vi "CR-字符串检测衬丝.vi"(8 "error in (no error)":errorcluster caption="错误输入（无错误）", 11 "名称或相对路径":string="Template Program") -> (0 "error in (no error) 2":errorcluster caption="错误输入（无错误）")   [LabVIEW 2017]
uses:
  Picture/SaveButtom.ctl
  <vilib>/vision/Measure.llb/Edge Options.ctl
  <vilib>/vision/Measure.llb/Edge Polarity.ctl
  <vilib>/userdefined/High Color/IMAQdx.ctl
  Global System.vi
  <vilib>/Utility/xml.llb/Write to XML File(string).vi
panel:
  in  "Line3 保护套基准ROI":bool
  in  "ROI获取 2":bool
  in  "line2 ROI获取":bool
  in  "line1 ROI获取":bool
  in  "相机选择":T1="cam4" caption="Session Out CCD3"
  in  "获取图像":bool
  in  "ROI获取":bool
  in  "保存图像":bool
  out "添加的路径":path
  in  "刷新":bool
  in  "测试按钮":bool
  in  "保存按钮":bool
  in  "Main":enum32{"主参数", "模板匹配参数 ", "ROI参数", "测试效果"}(tab)
  in  "衬丝检测基础参数":T2={"IsNorImage"=TRUE, "Exposure Values"=100289, "ImagePath"=path "C:/Users/hedongpo/Desktop/514-hdp/Alignment Assemble System/Test Picture/B/3.bmp"} caption="参数界面" {"Exposure Values" scale=0.0..200000.0}
  in  "CR- 衬丝检测参数":T6={"Settings (Clamp (Rake) 1)"={"Contrast"=65, "Filter width"=3, "Steepness"=6, "Subsampling Ratio"=9, "Show Search Area"=TRUE, "Show Search Lines"=FALSE, "Show Edges Found"=FALSE, "Show Result"=TRUE}, "Options (Find Straight Edge 1)"={"Search Direction"=0, "Edge Options"={"Edge Polarity"=1, "Kernel Size"=13, "Width"=1, "Minimum Edge Strength"=25.0, "Interpolation Type"=enum."Bilinear Fixed", "Data Processing Method"=enum."Average"}, "Show Search Area"=FALSE, "Show Search Lines"=FALSE, "Show Edges Found"=FALSE, "Show Result"=FALSE, "Search Area Color"=65280, "Search Lines Color"=255, "Edge Locations Color"=16776960, "Result Color"=16711680, "Overlay Group Name"=""}, "相对距离设定"={"上限"=925.0, "下限"=3.0}, "保护套角度"={"上限"=0.0, "下限"=0.0}, "保护套直径设定"={"上限"=0.0, "下限"=0.0}, "Edge Options (Edge Detector 1)"={"Edge Polarity"=0, "Kernel Size"=3, "Width"=3, "Minimum Edge Strength"=10.0, "Interpolation Type"=enum."Bilinear Fixed", "Data Processing Method"=enum."Average"}, "保护套标准位置"={"Start X"=0, "Start Y"=0, "End X"=0, "End Y"=0}} {"保护套标准位置"."Start X" scale=0.0..1024.0; "保护套标准位置"."End X" scale=0.0..1024.0; "Edge Options (Edge Detector 1)"."Edge Polarity" items=["All Edges", "Rising Edges", "Falling Edges"]; "Options (Find Straight Edge 1)"."Search Direction" items=["Left to Right", "Right to Left", "Top to Bottom", "Bottom to Top"]; "Options (Find Straight Edge 1)"."Edge Options"."Edge Polarity" items=["All Edges", "Rising Edges", "Falling Edges"]; "Options (Find Straight Edge 1)"."Edge Options"."Minimum Edge Strength" format="%.2f"; "Options (Find Straight Edge 1)"."Edge Options"."Width" step=2; "Options (Find Straight Edge 1)"."Edge Options"."Kernel Size" step=2}
  in  "CR- 衬丝检测ROI参数":T8 {"Line 2"."Start X" scale=0.0..1024.0; "Line 2"."End X" scale=0.0..1024.0; "clamp Rectangle"."Rotation" min=-90.0 max=90.0 step=1.0 format="%.2f"; "clamp Rectangle"."Left" scale=0.0..1024.0; "clamp Rectangle"."Right" scale=0.0..1024.0; "Line 1"."Start X" scale=0.0..1024.0; "Line 1"."End X" scale=0.0..1024.0; "find straight edge Rectangle"."Rotation" min=-90.0 max=90.0 step=1.0 format="%.2f"; "find straight edge Rectangle"."Left" scale=0.0..1024.0; "find straight edge Rectangle"."Right" scale=0.0..1024.0}
  out "保护套距离":bool
  out "原始图像":T9(plugin-control)
  out "Distance":sgl format="%.2f"
  out "衬丝有无":bool
  out "保护套与基准位置差异":sgl
  out "保护套直径":sgl
  out "路径输出":path
  in  "Vision Paramter Save Buttom":T10
  out "system time":string
  in  "取消按钮":bool
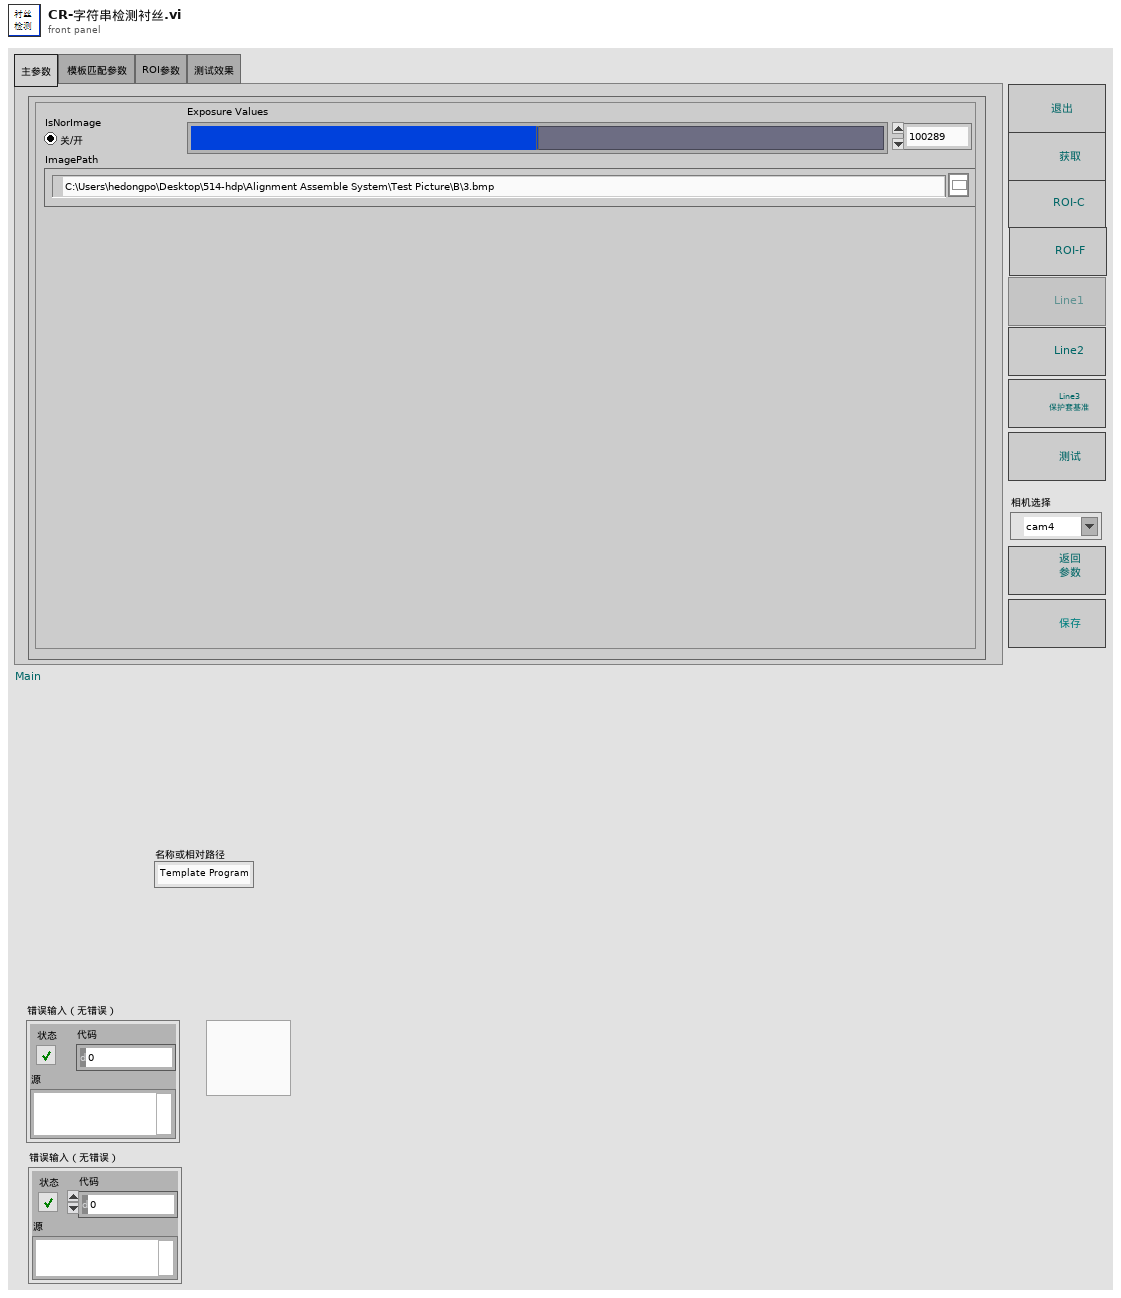
[diagram p1: front panel]
types:
  T1 = typedef "IMAQdx.ctl" = refnum<k21>
  T2 = cluster{"IsNorImage":bool, "Exposure Values":u32, "ImagePath":path}
  T3 = typedef "Edge Options.ctl" = cluster{"Edge Polarity":T4, "Kernel Size":u32, "Width":u32, "Minimum Edge Strength":sgl, "Interpolation Type":enum32{"Zero Order", "Bilinear", "Quadratic", "Cubic", "Bilinear Fixed"}, "Data Processing Method":enum32{"Average", "Median"}}
  T4 = typedef "Edge Polarity.ctl" = u32
  T5 = typedef "IMAQ Line" = cluster{"Start X":i32, "Start Y":i32, "End X":i32, "End Y":i32}
  T6 = cluster{"Settings (Clamp (Rake) 1)":cluster{"Contrast":i32, "Filter width":i32, "Steepness":i32, "Subsampling Ratio":u32, "Show Search Area":bool, "Show Search Lines":bool, "Show Edges Found":bool, "Show Result":bool}, "Options (Find Straight Edge 1)":cluster{"Search Direction":u32, "Edge Options":T3, "Show Search Area":bool, "Show Search Lines":bool, "Show Edges Found":bool, "Show Result":bool, "Search Area Color":u32, "Search Lines Color":u32, "Edge Locations Color":u32, "Result Color":u32, "Overlay Group Name":string}, "相对距离设定":cluster{"上限":dbl, "下限":dbl}, "保护套角度":cluster{"上限":dbl, "下限":dbl}, "保护套直径设定":cluster{"上限":dbl, "下限":dbl}, "Edge Options (Edge Detector 1)":cluster{"Edge Polarity":u32, "Kernel Size":u32, "Width":u32, "Minimum Edge Strength":sgl, "Interpolation Type":enum32{"Zero Order", "Bilinear", "Quadratic", "Cubic", "Bilinear Fixed"}, "Data Processing Method":enum32{"Average", "Median"}}, "保护套标准位置":T5}
  T7 = typedef "IMAQ Rectangle" = cluster{"Left":i32, "Top":i32, "Right":i32, "Bottom":i32, "Rotation":dbl}
  T8 = cluster{"find straight edge Rectangle":T7, "Line 1":T5, "clamp Rectangle ":T7, "Line 2":T5}
  T9 = typedef "IMAQ Image.ctl" = refnum<image>
  T10 = typedef "SaveButtom.ctl" = bool
  T11 = cluster{"index":i32, "this vi":refnum<vi>, "error out":errorcluster}
  T12 = cluster{"master data":string, "priority":u16, "secondary data":string[]}
  T13 = cluster{"case name":string[], "queue array":refnum<queue>[]}
  T14 = cluster{"Settings (Clamp (Rake) 1)":cluster{"Contrast":i32, "Filter width":i32, "Steepness":i32, "Subsampling Ratio":u32, "Show Search Area":bool, "Show Search Lines":bool, "Show Edges Found":bool, "Show Result":bool}, "Options (Find Straight Edge 1)":cluster{"Search Direction":u32, "Edge Options":T3, "Show Search Area":bool, "Show Search Lines":bool, "Show Edges Found":bool, "Show Result":bool, "Search Area Color":u32, "Search Lines Color":u32, "Edge Locations Color":u32, "Result Color":u32, "Overlay Group Name":string}, "相对距离设定":cluster{"上限":dbl, "下限":dbl}, "衬丝直径设定":cluster{"上限":dbl, "下限":dbl}, "保护套直径设定":cluster{"上限":dbl, "下限":dbl}, "Edge Options (Edge Detector 1)":cluster{"Edge Polarity":u32, "Kernel Size":u32, "Width":u32, "Minimum Edge Strength":sgl, "Interpolation Type":enum32{"Zero Order", "Bilinear", "Quadratic", "Cubic", "Bilinear Fixed"}, "Data Processing Method":enum32{"Average", "Median"}}, "保护套标准位置":T5}
  T15 = cluster{"Global Rectangle":i32[], "Contours":cluster{"Contour Type":u32, "ROI Type":u32, "Points":i32[]}[]}
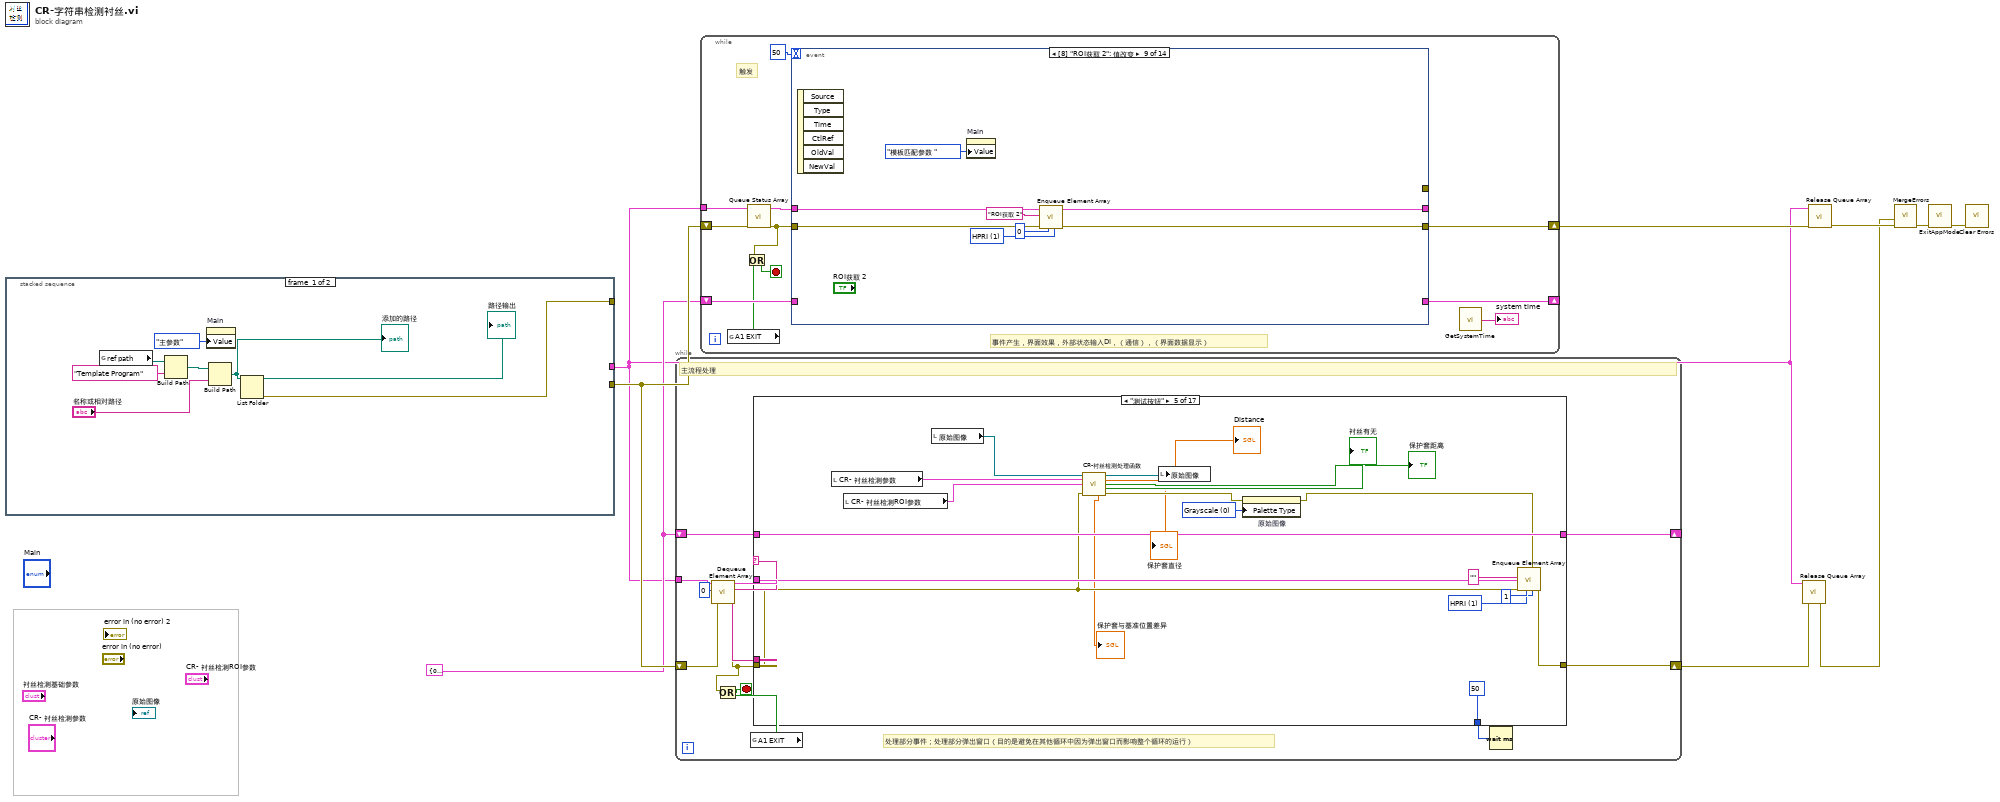
[diagram p0: block diagram]
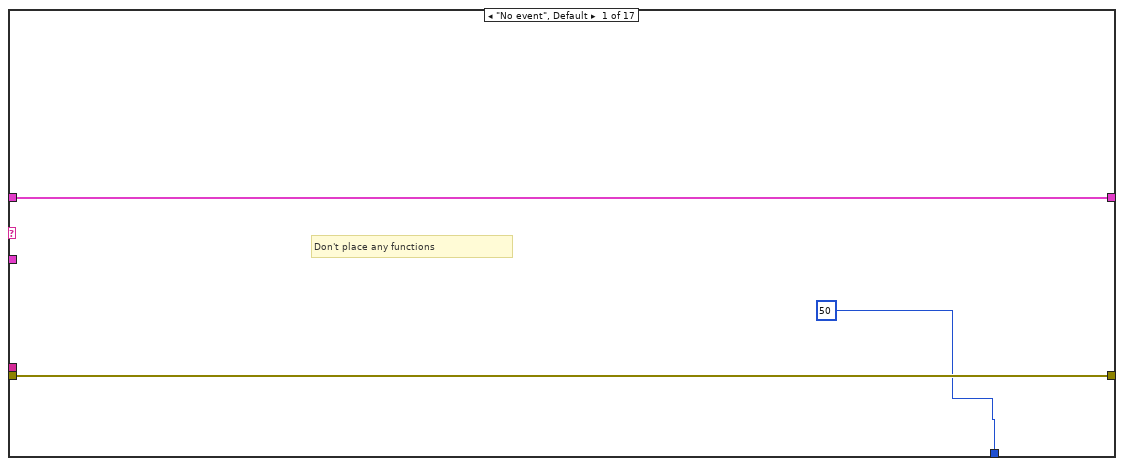
[diagram p2: hidden frame]
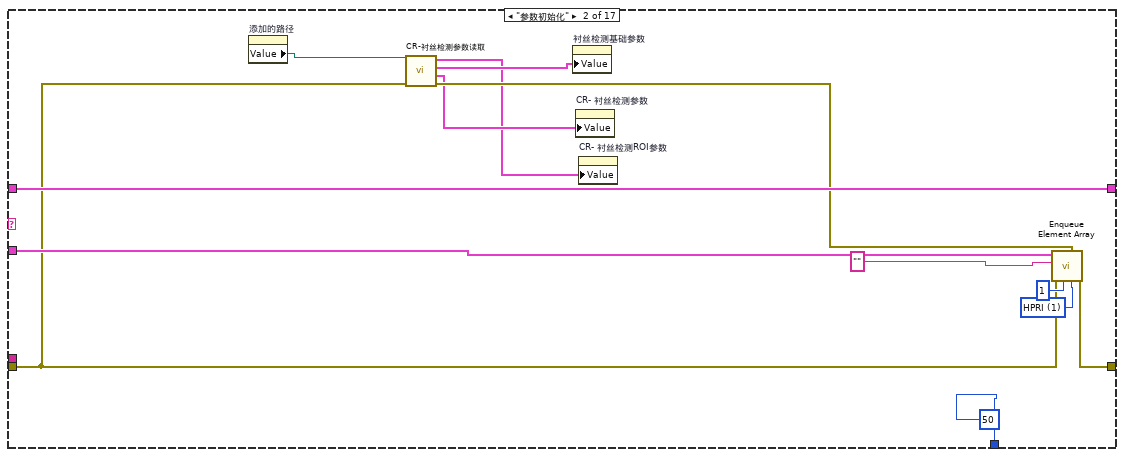
[diagram p3: hidden frame]
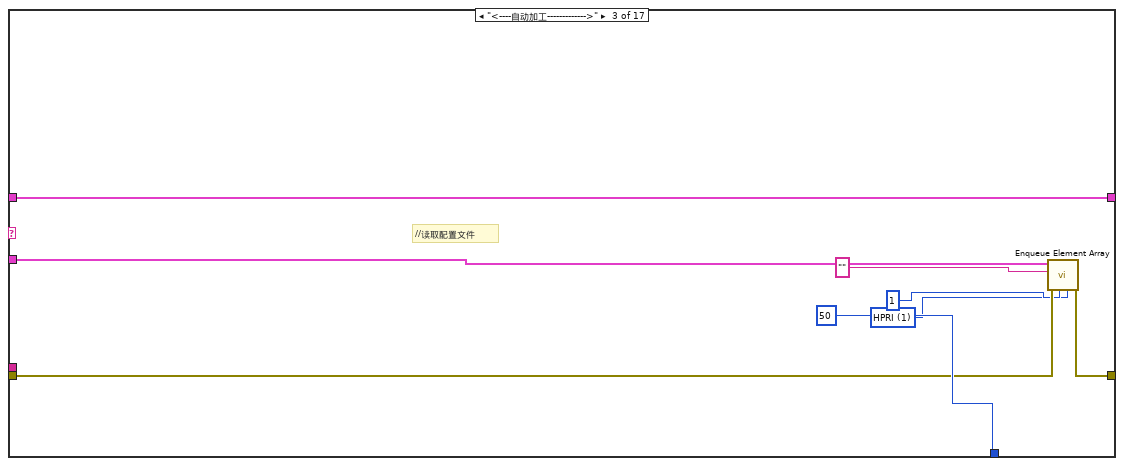
[diagram p4: hidden frame]
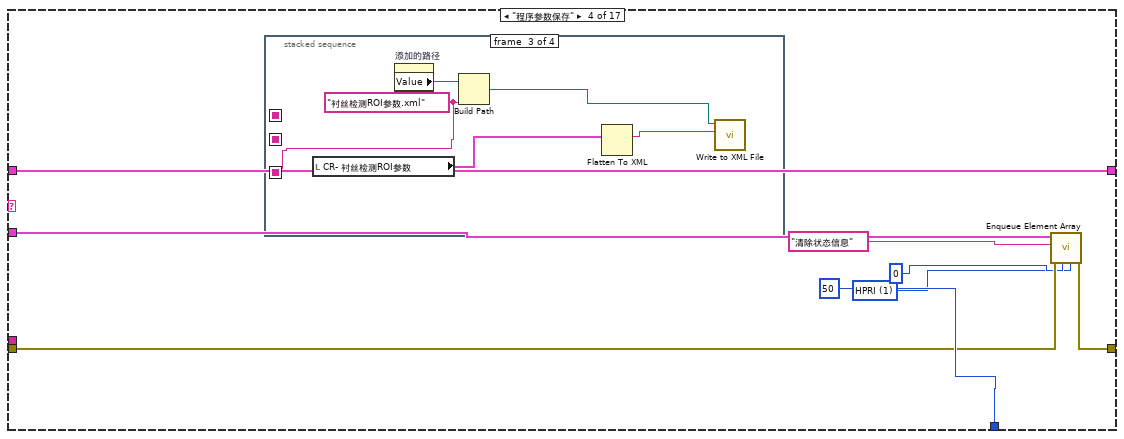
[diagram p5: hidden frame]
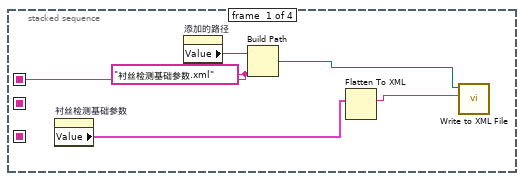
[diagram p6: hidden frame]
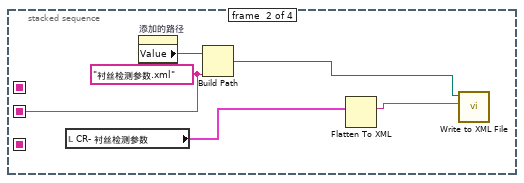
[diagram p7: hidden frame]
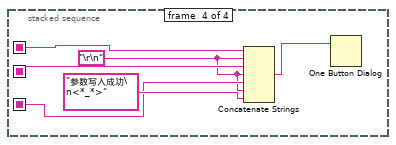
[diagram p8: hidden frame]
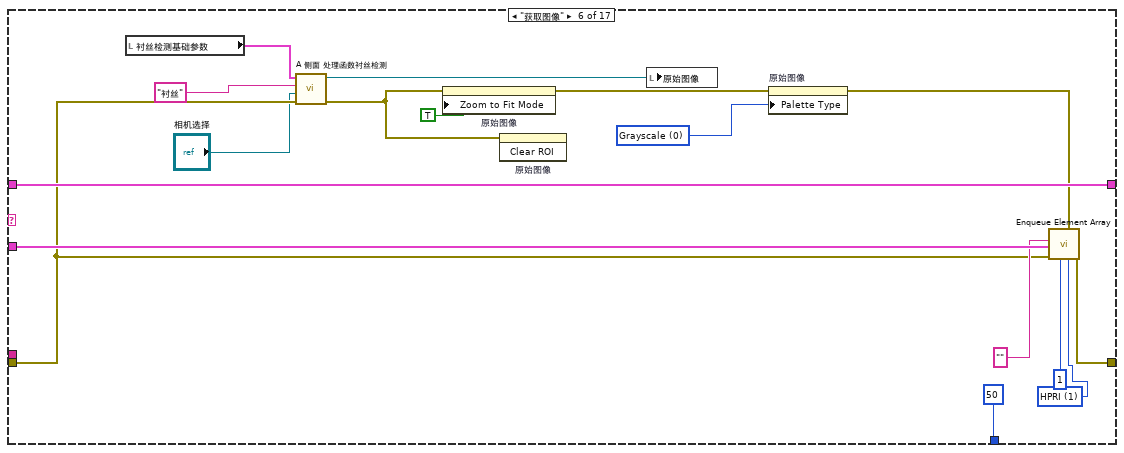
[diagram p9: hidden frame]
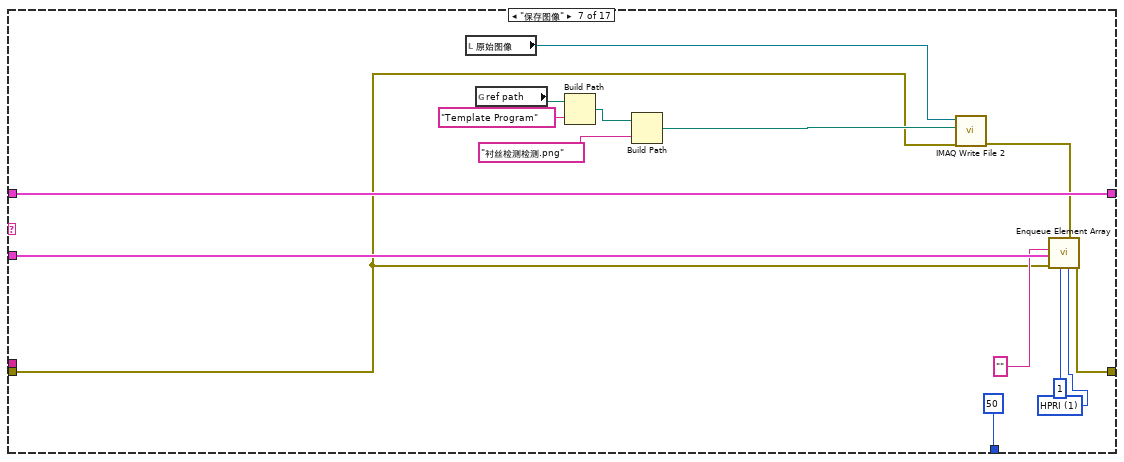
[diagram p10: hidden frame]
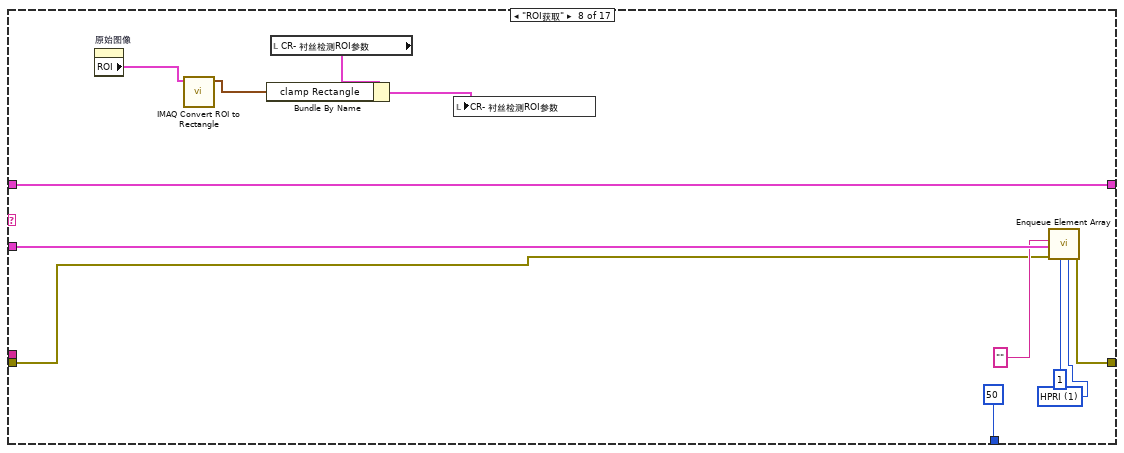
[diagram p11: hidden frame]
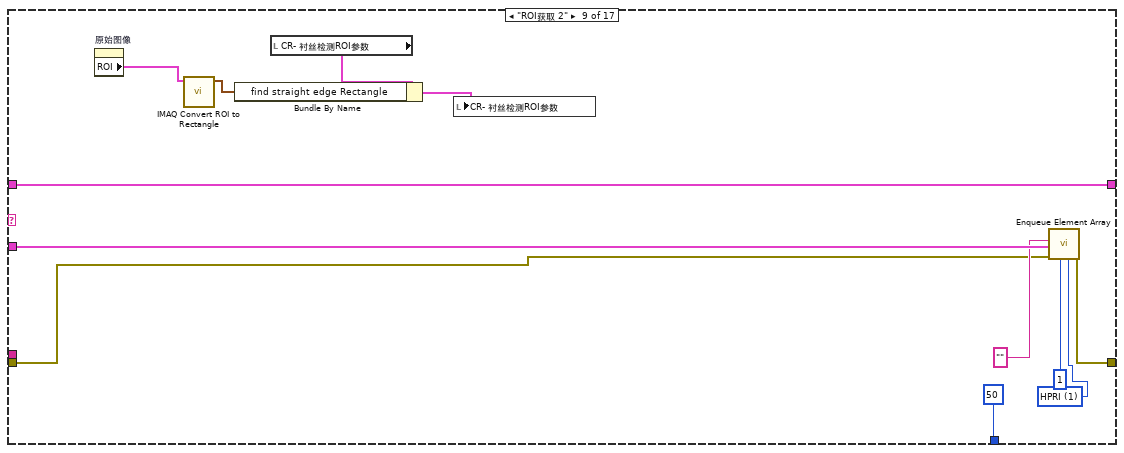
[diagram p12: hidden frame]
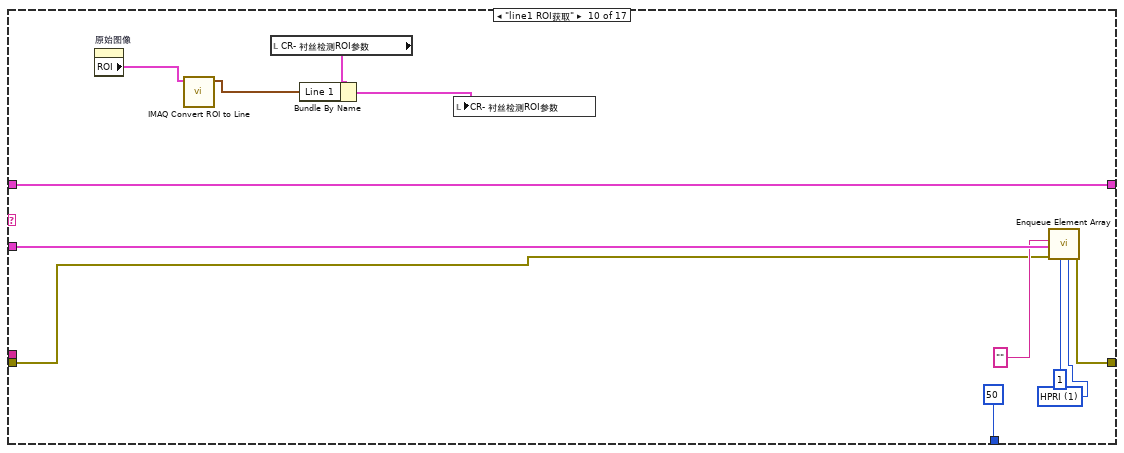
[diagram p13: hidden frame]
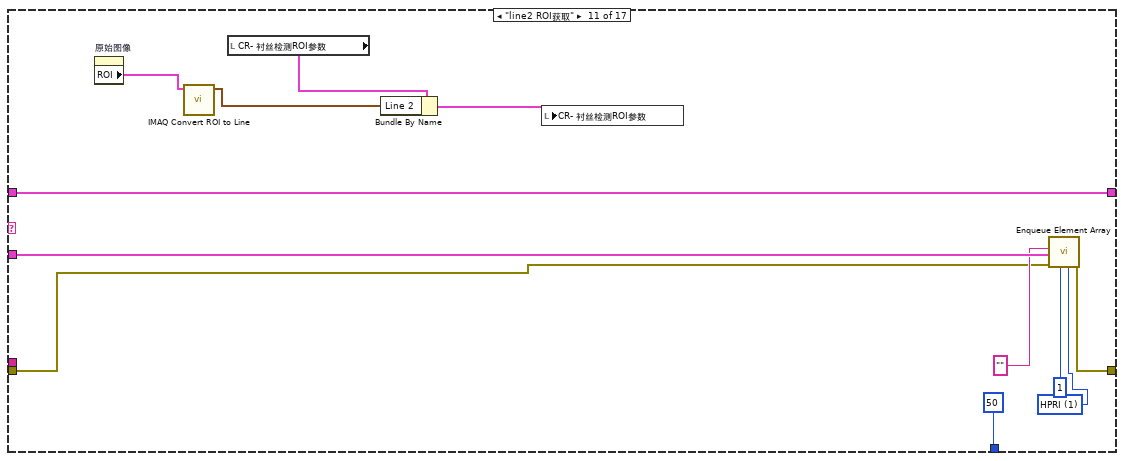
[diagram p14: hidden frame]
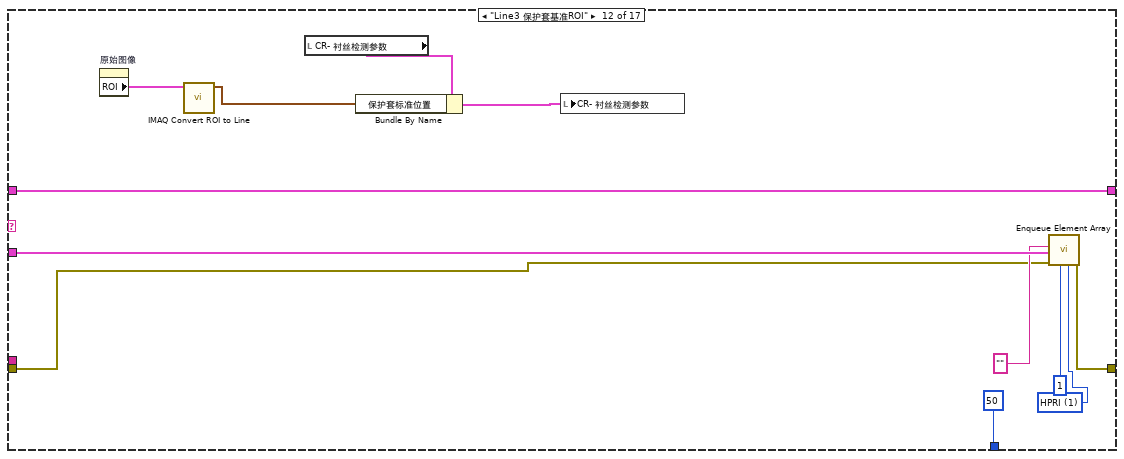
[diagram p15: hidden frame]
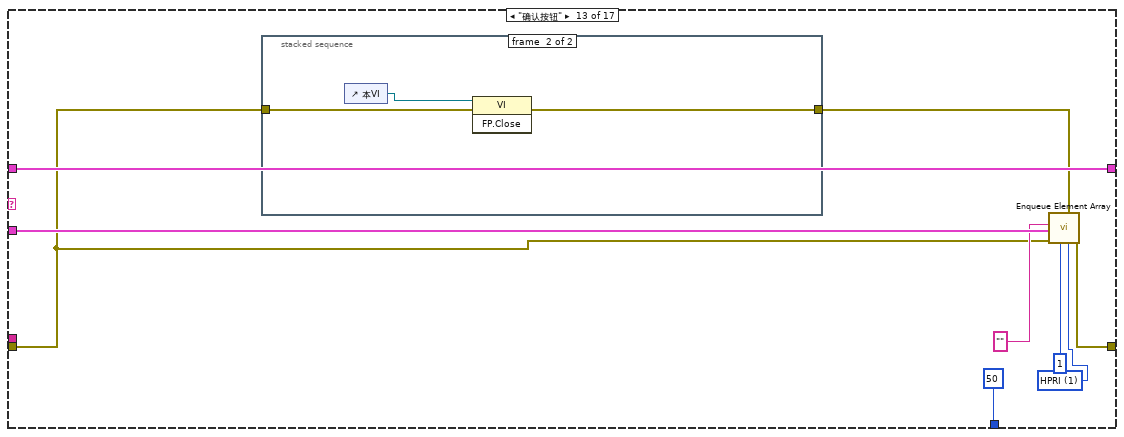
[diagram p16: hidden frame]
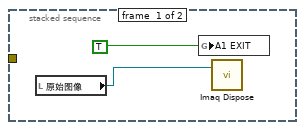
[diagram p17: hidden frame]
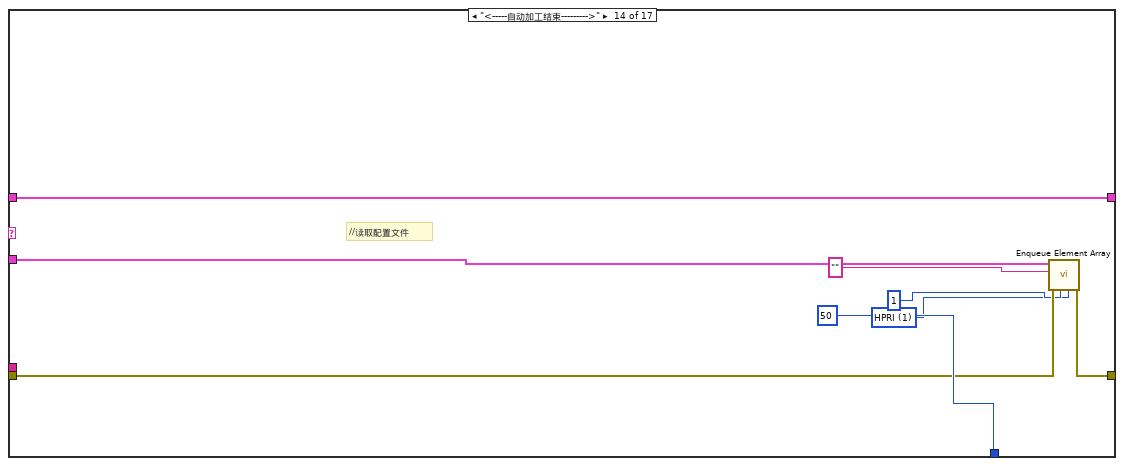
[diagram p18: hidden frame]
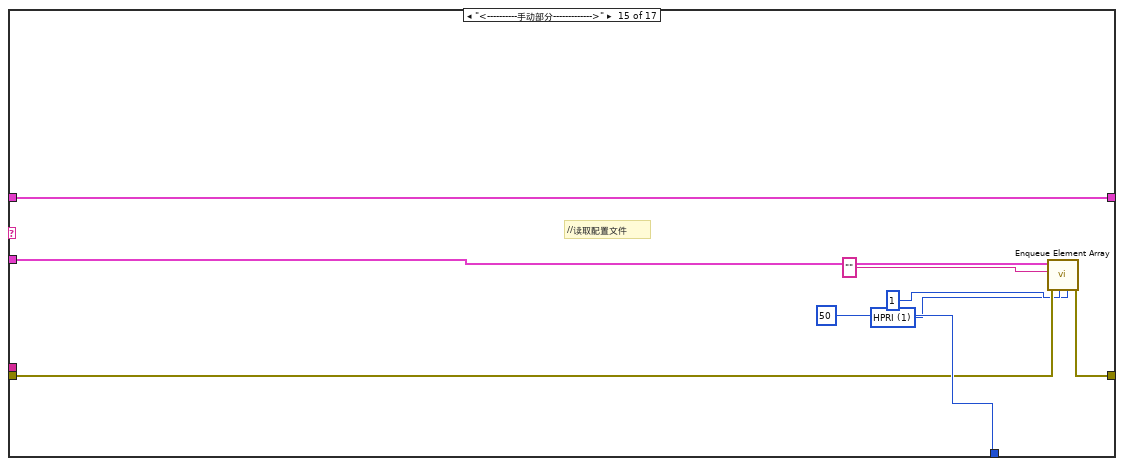
[diagram p19: hidden frame]
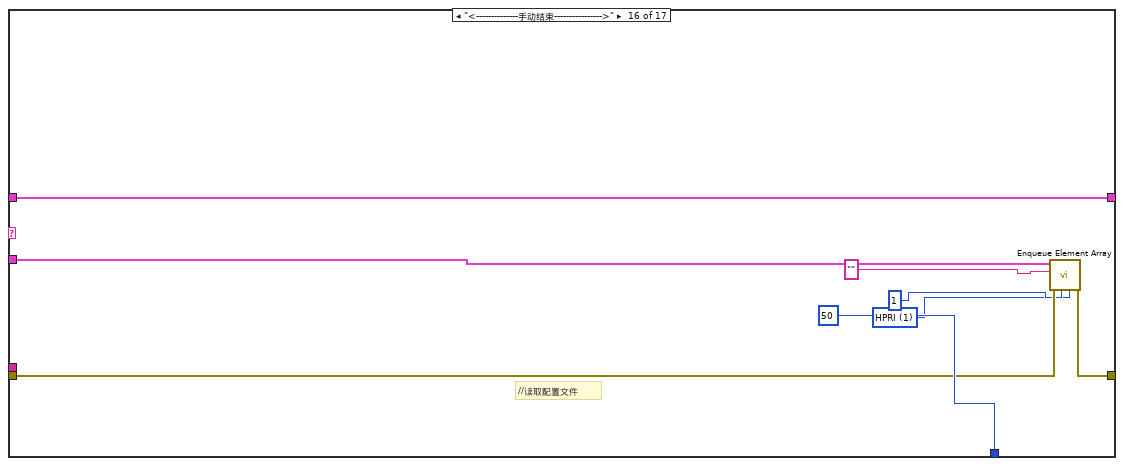
[diagram p20: hidden frame]
diagram:
  w4 = T11 {"index"=0, "this vi"=refnum, "error out"={"status"=FALSE, "code"=0, "source"=""}} ("parameter buffer")
  n1 = stacked-sequence {
    tunnel: [w15 _] -> _
    tunnel: [_ w19] -> w5
    tunnel: [_ w18] -> w1
    frame #0 {
      n2 = global read "Global System.vi" "ref path"() -> (w13:path)
      n3 = Build Path(base path=w13, name or relative path="Template Program" ("名称或相对路径")) -> (appended path=w11:path)
      n4 = property on="Main" class="TabCtl (严格)"("Value"=enum32{"主参数", "模板匹配参数 ", "ROI参数", "测试效果"}."主参数" ("Main")) -> ()  [unwired: 2 in, 2 out]
      n5 = Build Path(base path=w11, name or relative path="名称或相对路径") -> (appended path=w17:path)
      "添加的路径" <- w17
      n6 = List Folder(path=w17) -> (path out=→"路径输出":path, error out=w15:errorcluster)  [unwired: 3 in, 2 out]
    }
    frame #1 {
      w27 = string[] ["comm queue1", "data queue 11", "data queue 12", "data queue 13", "data queue 14"]  # queue name
      w28 = 4  # queue num
      w29 = T12 {"master data"="", "priority"=0, "secondary data"=[]}  # element data type
      n7 = call "Obtain Queue Array.vi"("queue name"=w27, "element data type"=w29, "queue num"=w28) -> ("error out"=w23:errorcluster, "queue out"=w24:T13)  [unwired: 2 in, 1 out]
      n8 = call "Enqueue Element Array.vi"("queue index"=0, "error in"=w23, "master data"="参数初始化", "queue in"=w24) -> ("error out"=w22:errorcluster, "queue out"=w21:T13)  [unwired: 6 in]
      n9 = disable-structure shown="启用" {
        disable-tunnel: w22 -> [w35 w36]
        disable-tunnel: w21 -> [w34 w37]
        disable-tunnel: "Loading Variable" ("master data") -> [w33 _]
        disable-tunnel: [w31 w36] -> w19
        disable-tunnel: [w30 w37] -> w18
        frame Disabled {
          n10 = call "Enqueue Element Array.vi"("queue index"=12, "error in"=w35, "master data"=w33, "queue in"=w34) -> ("error out"=w31:errorcluster, "queue out"=w30:T13)  [unwired: 6 in]
        }
        frame Enabled {
        }
      }
    }
  }
  n11 = while {
    shift-right: [w50] -> w3
    shift-left: w5 -> [w41]
    shift-right: [w47] -> _
    shift-left: w4 -> [w48]
    tunnel: w1 -> [w43]
    stop <- w38 stop-if-true
    # "处理部分事件；处理部分弹出窗口（目的是避免在其他循环中因为弹出窗口而影响整个循环的运行）"
    # "主流程处理"
    n12 = call "Dequeue Element Array.vi"("queue in"=w43, "queue index"=0, "error in"=w41) -> ("queue out"=w46:T13, "master data"=w45:string, "secondary data"=w44:string[], "error out"=w40:errorcluster)  [unwired: 2 in, 1 out]
    n13 = global read "Global System.vi" "A1 EXIT"() -> (w39:bool)
    n14 = Or(x=w40, y=w39) -> (x .or. y?=w38:bool)
    n15 = case shown="\"测试按钮\"" w45 {
      tunnel: w46 -> [_ w65 w73 w75 w122 w139 w154 w166 w178 w190 w202 w214 w223 w236 w244 w252 w258]
      tunnel: w40 -> [w52 w59 w69 w79 w116 w130 w142 w160 w172 w184 w196 w208 w217 w232 w240 w248 w255]
      tunnel: [w52 w64 w72 w81 w121 w138 w153 w165 w177 w189 w201 w213 w222 w235 w243 w251 w266] -> w50
      tunnel: [50 50 50 50 50 50 50 50 50 50 50 50 50 50 50 50 50] -> w49
      tunnel: w48 -> [w53 w60 w70 w76 w117 w134 w149 w161 w173 w185 w197 w209 w218 w233 w241 w249 w264]
      tunnel: [w53 w60 w70 w76 w117 w134 w149 w161 w173 w185 w197 w209 w218 w233 w241 w249 w264] -> w47
      tunnel: w44 -> [_ _ _ _ _ _ _ _ _ _ _ _ _ _ _ _ _]
      frame "No event", Default {
        # "Don't place any functions"
      }
      frame "参数初始化" {
        w61 = u16 1 items=["HPRI"=1, "LPRI"=0] ("priority")
        n16 = property on="添加的路径" class="Path"() -> ("Value"=w55:path)  [unwired: 2 in, 2 out]
        n17 = call "CR-衬丝检测参数读取.vi"("error in (no error)"=w59, "基路径"=w55) -> ("error out"=w58:errorcluster, "CR- 衬丝检测参数"=w56:T14, "衬丝检测基础参数"=w57:T2, "CR- 衬丝检测ROI参数"=w54:T8)  [unwired: 5 in]
        n18 = property on="衬丝检测基础参数" class="Clust (严格)"("Value"=w57) -> ()  [unwired: 2 in, 2 out]
        n19 = property on="CR- 衬丝检测参数" class="Clust (严格)"("Value"=w56) -> ()  [unwired: 2 in, 2 out]
        n20 = property on="CR- 衬丝检测ROI参数" class="Clust (严格)"("Value"=w54) -> ()  [unwired: 2 in, 2 out]
        n21 = call "Enqueue Element Array.vi"("priority"=w61, "device error in"=w58, "queue index"=1, "error in"=w59, "master data"="" ("Element 1"), "queue in"=w65) -> ("error out"=w64:errorcluster)  [unwired: 4 in, 1 out]
      }
      frame "<----自动加工------------->" {
        w67 = u16 1 items=["HPRI"=1, "LPRI"=0] ("priority")
        # "//读取配置文件"
        n22 = call "Enqueue Element Array.vi"("priority"=w67, "queue index"=1, "error in"=w69, "master data"="" ("Element 1"), "queue in"=w73) -> ("error out"=w72:errorcluster)  [unwired: 5 in, 1 out]
      }
      frame "程序参数保存" {
        w77 = u16 1 items=["HPRI"=1, "LPRI"=0] ("priority")
        n23 = stacked-sequence {
          seq-local: [w83 _ _ _] -> [_ _ _ w102]
          seq-local: [_ w92 _ _] -> [_ _ _ w100]
          seq-local: [_ _ w93 _] -> [_ _ _ w99]
          frame #0 {
            w83 = "衬丝检测基础参数.xml" ("名称或相对路径")
            n24 = property on="衬丝检测基础参数" class="Clust (严格)"() -> ("Value"=w86:T2)  [unwired: 2 in, 2 out]
            n25 = property on="添加的路径" class="Path"() -> ("Value"=w87:path)  [unwired: 2 in, 2 out]
            n26 = Build Path(base path=w87, name or relative path=w83) -> (appended path=w84:path)
            n27 = Flatten To XML(anything=w86) -> (xml string=w85:string)
            n28 = call-poly <vilib>:"Write to XML File.vi"("XML Input"=w85, "XML File Path"=w84) -> ()  [unwired: 7 in, 3 out]
          }
          frame #1 {
            w92 = "衬丝检测参数.xml" ("名称或相对路径")
            n29 = local read "CR- 衬丝检测参数"() -> (w88:T6)
            n30 = property on="添加的路径" class="Path"() -> ("Value"=w91:path)  [unwired: 2 in, 2 out]
            n31 = Build Path(base path=w91, name or relative path=w92) -> (appended path=w89:path)
            n32 = Flatten To XML(anything=w88) -> (xml string=w90:string)
            n33 = call-poly <vilib>:"Write to XML File.vi"("XML Input"=w90, "XML File Path"=w89) -> ()  [unwired: 7 in, 3 out]
          }
          frame #2 {
            w93 = "衬丝检测ROI参数.xml" ("名称或相对路径")
            n34 = local read "CR- 衬丝检测ROI参数"() -> (w94:T8)
            n35 = property on="添加的路径" class="Path"() -> ("Value"=w97:path)  [unwired: 2 in, 2 out]
            n36 = Build Path(base path=w97, name or relative path=w93) -> (appended path=w95:path)
            n37 = Flatten To XML(anything=w94) -> (xml string=w96:string)
            n38 = call-poly <vilib>:"Write to XML File.vi"("XML Input"=w96, "XML File Path"=w95) -> ()  [unwired: 7 in, 3 out]
          }
          frame #3 {
            w98 = "\r\n"
            n39 = Concatenate Strings(w102, w98, w100, w98, w99, w98, "参数写入成功\n<*_*>" ("消息")) -> (w101:string)
            n40 = One Button Dialog(message=w101) -> ()  [unwired: 1 in, 1 out]
          }
        }
        n41 = call "Enqueue Element Array.vi"("priority"=w77, "queue index"=0, "error in"=w79, "master data"="清除状态信息" ("Element 1"), "queue in"=w75) -> ("error out"=w81:errorcluster)  [unwired: 5 in, 1 out]
      }
      frame "测试按钮" {
        w113 = u32 0 items=["Grayscale", "Binary", "Gradient", "Rainbow", "Temperature", "User Defined", "Binary 16 Bit", "Gradient 16 Bit", "Rainbow 16 Bit", "Temperature 16 Bit", "User Defined 16 Bit"] ("Palette:Palette Type")
        w118 = u16 1 items=["HPRI"=1, "LPRI"=0] ("priority")
        n42 = local read "CR- 衬丝检测参数"() -> (w109:T6)
        n43 = local read "CR- 衬丝检测ROI参数"() -> (w105:T8)
        n44 = local read "原始图像"() -> (w114:T9)
        n45 = call "CR-衬丝检测处理函数.vi"("Image in"=w114, "CR- 衬丝检测参数"=w109, "CR- 衬丝检测ROI参数"=w105, "error in (no error)"=w116) -> ("Image out"=w115:T9, "Distance (Clamp (Rake) 1)"=→"Distance":sgl, "保护套距离"=→"保护套距离":bool, "衬丝有无"=→"衬丝有无":bool, "保护套直径"=→"保护套直径":sgl, "保护套与基准位置差值"=→"保护套与基准位置差异":sgl, "error out"=w112:errorcluster)  [unwired: 5 in]
        n46 = local write "原始图像"(w115) -> ()
        n47 = property on="原始图像" class="ImageControl"(error in=w112, "Palette Type"=w113) -> (error out=w111:errorcluster)  [unwired: 1 in, 1 out]
        n48 = call "Enqueue Element Array.vi"("priority"=w118, "device error in"=w111, "queue index"=1, "error in"=w116, "master data"="" ("Element 1"), "queue in"=w122) -> ("error out"=w121:errorcluster)  [unwired: 4 in, 1 out]
      }
      frame "获取图像" {
        w127 = u32 0 items=["Grayscale", "Binary", "Gradient", "Rainbow", "Temperature", "User Defined", "Binary 16 Bit", "Gradient 16 Bit", "Rainbow 16 Bit", "Temperature 16 Bit", "User Defined 16 Bit"] ("Palette:Palette Type")
        w135 = u16 1 items=["HPRI"=1, "LPRI"=0] ("priority")
        n49 = local read "衬丝检测基础参数"() -> (w132:T2)
        n50 = call "A 侧面 处理函数衬丝检测.vi"("error in (no error)"=w130, "Session in"="相机选择", "Image Name"="衬丝", "CR-检测基础参数"=w132) -> ("error out"=w128:errorcluster, "Image out"=w131:T9)  [unwired: 4 in, 2 out]
        n51 = property on="原始图像" class="ImageControl"(error in=w128, "Zoom to Fit Mode"=TRUE) -> (error out=w126:errorcluster)  [unwired: 1 in, 1 out]
        n52 = invoke on="原始图像" class="ImageControl" method="Clear ROI"(error in=w128) -> ()  [unwired: 2 in, 3 out]
        n53 = local write "原始图像"(w131) -> ()
        n54 = property on="原始图像" class="ImageControl"(error in=w126, "Palette Type"=w127) -> (error out=w125:errorcluster)  [unwired: 1 in, 1 out]
        n55 = call "Enqueue Element Array.vi"("priority"=w135, "device error in"=w125, "queue index"=1, "error in"=w130, "master data"="" ("Element 1"), "queue in"=w139) -> ("error out"=w138:errorcluster)  [unwired: 4 in, 1 out]
      }
      frame "保存图像" {
        w150 = u16 1 items=["HPRI"=1, "LPRI"=0] ("priority")
        n56 = local read "原始图像"() -> (w141:T9)
        n57 = global read "Global System.vi" "ref path"() -> (w148:path)
        n58 = Build Path(base path=w148, name or relative path="Template Program" ("名称或相对路径")) -> (appended path=w146:path)
        n59 = Build Path(base path=w146, name or relative path="衬丝检测检测.png" ("名称或相对路径")) -> (appended path=w144:path)
        n60 = call-poly "IMAQ Write File 2"("error in (no error)"=w142, "File Path"=w144, "Image"=w141) -> ("error out"=w143:errorcluster)  [unwired: 7 in, 1 out]
        n61 = call "Enqueue Element Array.vi"("priority"=w150, "device error in"=w143, "queue index"=1, "error in"=w142, "master data"="" ("Element 1"), "queue in"=w154) -> ("error out"=w153:errorcluster)  [unwired: 4 in, 1 out]
      }
      frame "ROI获取" {
        w162 = u16 1 items=["HPRI"=1, "LPRI"=0] ("priority")
        n62 = property on="原始图像" class="ImageControl"() -> ("ROI"=w157:T15)  [unwired: 2 in, 2 out]
        n63 = call "IMAQ Convert ROI to Rectangle"("ROI Descriptor"=w157) -> ("Rectangle"=w156:T7)  [unwired: 8 in, 1 out]
        n64 = local read "CR- 衬丝检测ROI参数"() -> (w159:T8)
        n65 = Bundle By Name(cluster=w159, "clamp Rectangle"=w156) -> (w158:T8)
        n66 = local write "CR- 衬丝检测ROI参数"(w158) -> ()
        n67 = call "Enqueue Element Array.vi"("priority"=w162, "queue index"=1, "error in"=w160, "master data"="" ("Element 1"), "queue in"=w166) -> ("error out"=w165:errorcluster)  [unwired: 5 in, 1 out]
      }
      frame "ROI获取 2" {
        w174 = u16 1 items=["HPRI"=1, "LPRI"=0] ("priority")
        n68 = property on="原始图像" class="ImageControl"() -> ("ROI"=w169:T15)  [unwired: 2 in, 2 out]
        n69 = call "IMAQ Convert ROI to Rectangle"("ROI Descriptor"=w169) -> ("Rectangle"=w168:T7)  [unwired: 8 in, 1 out]
        n70 = local read "CR- 衬丝检测ROI参数"() -> (w171:T8)
        n71 = Bundle By Name(cluster=w171, "find straight edge Rectangle"=w168) -> (w170:T8)
        n72 = local write "CR- 衬丝检测ROI参数"(w170) -> ()
        n73 = call "Enqueue Element Array.vi"("priority"=w174, "queue index"=1, "error in"=w172, "master data"="" ("Element 1"), "queue in"=w178) -> ("error out"=w177:errorcluster)  [unwired: 5 in, 1 out]
      }
      frame "line1 ROI获取" {
        w186 = u16 1 items=["HPRI"=1, "LPRI"=0] ("priority")
        n74 = property on="原始图像" class="ImageControl"() -> ("ROI"=w181:T15)  [unwired: 2 in, 2 out]
        n75 = call "IMAQ Convert ROI to Line"("ROI Descriptor"=w181) -> ("Line"=w180:T5)  [unwired: 8 in, 1 out]
        n76 = local read "CR- 衬丝检测ROI参数"() -> (w183:T8)
        n77 = Bundle By Name(cluster=w183, "Line 1"=w180) -> (w182:T8)
        n78 = local write "CR- 衬丝检测ROI参数"(w182) -> ()
        n79 = call "Enqueue Element Array.vi"("priority"=w186, "queue index"=1, "error in"=w184, "master data"="" ("Element 1"), "queue in"=w190) -> ("error out"=w189:errorcluster)  [unwired: 5 in, 1 out]
      }
      frame "line2 ROI获取" {
        w198 = u16 1 items=["HPRI"=1, "LPRI"=0] ("priority")
        n80 = property on="原始图像" class="ImageControl"() -> ("ROI"=w193:T15)  [unwired: 2 in, 2 out]
        n81 = call "IMAQ Convert ROI to Line"("ROI Descriptor"=w193) -> ("Line"=w192:T5)  [unwired: 8 in, 1 out]
        n82 = local read "CR- 衬丝检测ROI参数"() -> (w195:T8)
        n83 = Bundle By Name(cluster=w195, "Line 2"=w192) -> (w194:T8)
        n84 = local write "CR- 衬丝检测ROI参数"(w194) -> ()
        n85 = call "Enqueue Element Array.vi"("priority"=w198, "queue index"=1, "error in"=w196, "master data"="" ("Element 1"), "queue in"=w202) -> ("error out"=w201:errorcluster)  [unwired: 5 in, 1 out]
      }
      frame "Line3 保护套基准ROI" {
        w210 = u16 1 items=["HPRI"=1, "LPRI"=0] ("priority")
        n86 = property on="原始图像" class="ImageControl"() -> ("ROI"=w207:T15)  [unwired: 2 in, 2 out]
        n87 = call "IMAQ Convert ROI to Line"("ROI Descriptor"=w207) -> ("Line"=w206:T5)  [unwired: 8 in, 1 out]
        n88 = local read "CR- 衬丝检测参数"() -> (w204:T6)
        n89 = Bundle By Name(cluster=w204, "保护套标准位置"=w206) -> (w205:T6)
        n90 = local write "CR- 衬丝检测参数"(w205) -> ()
        n91 = call "Enqueue Element Array.vi"("priority"=w210, "queue index"=1, "error in"=w208, "master data"="" ("Element 1"), "queue in"=w214) -> ("error out"=w213:errorcluster)  [unwired: 5 in, 1 out]
      }
      frame "确认按钮" {
        w219 = u16 1 items=["HPRI"=1, "LPRI"=0] ("priority")
        n92 = stacked-sequence {
          tunnel: w217 -> [_ w228]
          tunnel: [_ w227] -> w216
          frame #0 {
            n93 = local read "原始图像"() -> (w225:T9)
            n94 = global write "Global System.vi" "A1 EXIT"(TRUE ("EXIT")) -> ()
            n95 = call "Imaq Dispose"("Image"=w225) -> ()  [unwired: 5 in, 1 out]
          }
          frame #1 {
            n96 = control-ref of="本VI"() -> (w229:refnum<vi>)
            n97 = invoke class="VI" method="FP.Close"(reference=w229, error in=w228) -> (error out=w227:errorcluster)  [unwired: 1 in, 2 out]
          }
        }
        n98 = call "Enqueue Element Array.vi"("priority"=w219, "device error in"=w216, "queue index"=1, "error in"=w217, "master data"="" ("Element 1"), "queue in"=w223) -> ("error out"=w222:errorcluster)  [unwired: 4 in, 1 out]
      }
      frame "<-----自动加工结束--------->" {
        w230 = u16 1 items=["HPRI"=1, "LPRI"=0] ("priority")
        # "//读取配置文件"
        n99 = call "Enqueue Element Array.vi"("priority"=w230, "queue index"=1, "error in"=w232, "master data"="" ("Element 1"), "queue in"=w236) -> ("error out"=w235:errorcluster)  [unwired: 5 in, 1 out]
      }
      frame "<----------手动部分------------->" {
        w238 = u16 1 items=["HPRI"=1, "LPRI"=0] ("priority")
        # "//读取配置文件"
        n100 = call "Enqueue Element Array.vi"("priority"=w238, "queue index"=1, "error in"=w240, "master data"="" ("Element 1"), "queue in"=w244) -> ("error out"=w243:errorcluster)  [unwired: 5 in, 1 out]
      }
      frame "<--------------手动结束---------------->" {
        w246 = u16 1 items=["HPRI"=1, "LPRI"=0] ("priority")
        # "//读取配置文件"
        n101 = call "Enqueue Element Array.vi"("priority"=w246, "queue index"=1, "error in"=w248, "master data"="" ("Element 1"), "queue in"=w252) -> ("error out"=w251:errorcluster)  [unwired: 5 in, 1 out]
      }
      frame "*Emergency alarm" {
        w261 = u16 1 items=["HPRI"=1, "LPRI"=0] ("priority")
        w262 = u16 1 items=["HPRI"=1, "LPRI"=0] ("priority")
        # "发出处理急停信号的命令"
        # "发出处理急停信号的命令"
        n102 = call "Enqueue Element Array.vi"("priority"=w261, "queue index"=0, "error in"=w255, "master data"="" ("Element 1"), "queue in"=w258) -> ("error out"=w256:errorcluster, "queue out"=w257:T13)  [unwired: 5 in]
        n103 = call "SetTestInfoIndex.vi"("test info index"=13) -> ()
        n104 = call "Enqueue Element Array.vi"("priority"=w262, "queue index"=1, "error in"=w256, "master data"="" ("Element 1"), "queue in"=w257) -> ("error out"=w266:errorcluster)  [unwired: 5 in, 1 out]
      }
    }
    n105 = Wait (ms)(milliseconds to wait=w49) -> ()  [unwired: 1 out]
  }
  n106 = while {
    shift-right: [w271] -> w6
    shift-left: w5 -> [w275]
    shift-right: [w273] -> _
    shift-left: w4 -> [w274]
    tunnel: w1 -> [w277]
    stop <- w268 stop-if-true
    # "触发"
    # "事件产生，界面效果，外部状态输入DI，（通信），（界面数据显示）"
    n107 = global read "Global System.vi" "A1 EXIT"() -> (w269:bool)
    n108 = call "Queue Status Array.vi"("error in (no error)"=w275, "queue in"=w277) -> ("error out"=w270:errorcluster, "queue out"=w272:T13)  [unwired: 4 in]
    n109 = Or(x=w270, y=w269) -> (x .or. y?=w268:bool)
    n110 = event shown="[8] \"ROI获取 2\": 值改变" {
      selector: _ -> [_ _ _ _ _ _ _ _ _ _ _ _ _ _]
      dyn-events: _ -> [_ _ _ _ _ _ _ _ _ _ _ _ _ _]
      timeout: 50 -> [_ _ _ _ _ _ _ _ _ _ _ _ _ _]
      tunnel: w274 -> [w282 w290 _ _ _ _ _ _ _ _ _ _ _ _]
      tunnel: [w282 w290 _ _ _ _ _ _ _ _ _ _ _ _] -> w273
      tunnel: [errorcluster {"status"=FALSE, "code"=0, "source"=""} ("error out") _ _ _ _ _ _ _ _ _ _ _ _ _] -> _
      tunnel: w272 -> [w280 w289 w295 w302 w309 w317 w324 w332 w340 w348 w356 w364 w372 w380]
      tunnel: w270 -> [w279 w288 w294 w301 w308 w316 w323 w331 w339 w347 w355 w363 w371 w379]
      tunnel: [w279 w287 w292 w299 w306 w314 w321 w329 w337 w345 w353 w361 w369 w377] -> w271
      tunnel: [w280 w286 w293 w300 w307 w315 w322 w330 w338 w346 w354 w362 w370 w378] -> _
      event Timeout {
        # "不要在事件结构里面放入\"弹出窗口\"这样的VI保证该循环畅通无阻。"
        n111 = event-data() -> ()  [unwired: 1 in, 1 out]
      }
      event Panel Close? {
        w284 = u16 1 items=["HPRI"=1, "LPRI"=0] ("priority")
        n112 = event-data() -> ()  [unwired: 1 in, 4 out]
        n113 = call "Enqueue Element Array.vi"("priority"=w284, "queue index"=0, "error in"=w288, "master data"="*Exit application", "queue in"=w289) -> ("error out"=w287:errorcluster, "queue out"=w286:T13)  [unwired: 5 in]
        n114 = event-data("Discard?"=TRUE) -> ()  [unwired: 1 in, 1 out]
      }
      event Value Change {
        w297 = u16 1 items=["HPRI"=1, "LPRI"=0] ("priority")
        n115 = event-data() -> ()  [unwired: 1 in, 6 out]
        n116 = call "Enqueue Element Array.vi"("priority"=w297, "queue index"=0, "error in"=w294, "master data"="Vision Paramter Save", "queue in"=w295) -> ("error out"=w292:errorcluster, "queue out"=w293:T13)  [unwired: 5 in]
      }
      event "取消按钮": Value Change {
        w304 = u16 1 items=["HPRI"=1, "LPRI"=0] ("priority")
        n117 = event-data() -> ()  [unwired: 1 in, 6 out]
        n118 = call "Enqueue Element Array.vi"("priority"=w304, "queue index"=0, "error in"=w301, "master data"="确认按钮", "queue in"=w302) -> ("error out"=w299:errorcluster, "queue out"=w300:T13)  [unwired: 5 in]
      }
      event "保存按钮": Value Change {
        w311 = u16 1 items=["HPRI"=1, "LPRI"=0] ("priority")
        n119 = event-data() -> ()  [unwired: 1 in, 6 out]
        n120 = call "Enqueue Element Array.vi"("priority"=w311, "queue index"=0, "error in"=w308, "master data"="程序参数保存", "queue in"=w309) -> ("error out"=w306:errorcluster, "queue out"=w307:T13)  [unwired: 5 in]
      }
      event "获取图像": Value Change {
        w319 = u16 1 items=["HPRI"=1, "LPRI"=0] ("priority")
        n121 = event-data() -> ()  [unwired: 1 in, 6 out]
        n122 = property on="Main" class="TabCtl (严格)"("Value"=enum32{"主参数", "模板匹配参数 ", "ROI参数", "测试效果"}."测试效果" ("Main")) -> ()  [unwired: 2 in, 2 out]
        n123 = call "Enqueue Element Array.vi"("priority"=w319, "queue index"=0, "error in"=w316, "master data"="获取图像", "queue in"=w317) -> ("error out"=w314:errorcluster, "queue out"=w315:T13)  [unwired: 5 in]
      }
      event "保存图像": Value Change {
        w326 = u16 1 items=["HPRI"=1, "LPRI"=0] ("priority")
        n124 = event-data() -> ()  [unwired: 1 in, 6 out]
        n125 = call "Enqueue Element Array.vi"("priority"=w326, "queue index"=0, "error in"=w323, "master data"="保存图像", "queue in"=w324) -> ("error out"=w321:errorcluster, "queue out"=w322:T13)  [unwired: 5 in]
      }
      event "ROI获取": Value Change {
        w334 = u16 1 items=["HPRI"=1, "LPRI"=0] ("priority")
        n126 = event-data() -> ()  [unwired: 1 in, 6 out]
        n127 = property on="Main" class="TabCtl (严格)"("Value"=enum32{"主参数", "模板匹配参数 ", "ROI参数", "测试效果"}."模板匹配参数 " ("Main")) -> ()  [unwired: 2 in, 2 out]
        n128 = call "Enqueue Element Array.vi"("priority"=w334, "queue index"=0, "error in"=w331, "master data"="ROI获取", "queue in"=w332) -> ("error out"=w329:errorcluster, "queue out"=w330:T13)  [unwired: 5 in]
      }
      event "ROI获取 2": Value Change {
        w342 = u16 1 items=["HPRI"=1, "LPRI"=0] ("priority")
        n129 = event-data() -> ()  [unwired: 1 in, 6 out]
        n130 = property on="Main" class="TabCtl (严格)"("Value"=enum32{"主参数", "模板匹配参数 ", "ROI参数", "测试效果"}."模板匹配参数 " ("Main")) -> ()  [unwired: 2 in, 2 out]
        n131 = call "Enqueue Element Array.vi"("priority"=w342, "queue index"=0, "error in"=w339, "master data"="ROI获取 2", "queue in"=w340) -> ("error out"=w337:errorcluster, "queue out"=w338:T13)  [unwired: 5 in]
      }
      event "Line3 保护套基准ROI": Value Change {
        w350 = u16 1 items=["HPRI"=1, "LPRI"=0] ("priority")
        n132 = event-data() -> ()  [unwired: 1 in, 6 out]
        n133 = property on="Main" class="TabCtl (严格)"("Value"=enum32{"主参数", "模板匹配参数 ", "ROI参数", "测试效果"}."模板匹配参数 " ("Main")) -> ()  [unwired: 2 in, 2 out]
        n134 = call "Enqueue Element Array.vi"("priority"=w350, "queue index"=0, "error in"=w347, "master data"="Line3 保护套基准ROI", "queue in"=w348) -> ("error out"=w345:errorcluster, "queue out"=w346:T13)  [unwired: 5 in]
      }
      event "line1 ROI获取": Value Change {
        w358 = u16 1 items=["HPRI"=1, "LPRI"=0] ("priority")
        n135 = event-data() -> ()  [unwired: 1 in, 6 out]
        n136 = property on="Main" class="TabCtl (严格)"("Value"=enum32{"主参数", "模板匹配参数 ", "ROI参数", "测试效果"}."模板匹配参数 " ("Main")) -> ()  [unwired: 2 in, 2 out]
        n137 = call "Enqueue Element Array.vi"("priority"=w358, "queue index"=0, "error in"=w355, "master data"="line1 ROI获取", "queue in"=w356) -> ("error out"=w353:errorcluster, "queue out"=w354:T13)  [unwired: 5 in]
      }
      event "line2 ROI获取": Value Change {
        w366 = u16 1 items=["HPRI"=1, "LPRI"=0] ("priority")
        n138 = event-data() -> ()  [unwired: 1 in, 6 out]
        n139 = call "Enqueue Element Array.vi"("priority"=w366, "queue index"=0, "error in"=w363, "master data"="line2 ROI获取", "queue in"=w364) -> ("error out"=w361:errorcluster, "queue out"=w362:T13)  [unwired: 5 in]
        n140 = property on="Main" class="TabCtl (严格)"("Value"=enum32{"主参数", "模板匹配参数 ", "ROI参数", "测试效果"}."模板匹配参数 " ("Main")) -> ()  [unwired: 2 in, 2 out]
      }
      event "测试按钮": Value Change {
        w374 = u16 1 items=["HPRI"=1, "LPRI"=0] ("priority")
        n141 = event-data() -> ()  [unwired: 1 in, 6 out]
        n142 = call "Enqueue Element Array.vi"("priority"=w374, "queue index"=0, "error in"=w371, "master data"="测试按钮", "queue in"=w372) -> ("error out"=w369:errorcluster, "queue out"=w370:T13)  [unwired: 5 in]
        n143 = property on="Main" class="TabCtl (严格)"("Value"=enum32{"主参数", "模板匹配参数 ", "ROI参数", "测试效果"}."测试效果" ("Main")) -> ()  [unwired: 2 in, 2 out]
      }
      event "刷新": Value Change {
        n144 = event-data() -> ()  [unwired: 1 in, 6 out]
        n145 = disable-structure shown="禁用" {
          disable-tunnel: w380 -> [w384 _]
          disable-tunnel: w379 -> [w383 _]
          disable-tunnel: [w382 _] -> w378
          disable-tunnel: [w381 _] -> w377
          frame Disabled {
            w386 = u16 1 items=["HPRI"=1, "LPRI"=0] ("priority")
            # "刷新"
            n146 = call "Enqueue Element Array.vi"("priority"=w386, "queue index"=0, "error in"=w383, "master data"="刷新", "queue in"=w384) -> ("error out"=w381:errorcluster, "queue out"=w382:T13)  [unwired: 5 in]
          }
          frame Enabled {
          }
        }
        n147 = property on="Main" class="TabCtl (严格)"("Value"=enum32{"主参数", "模板匹配参数 ", "ROI参数", "测试效果"}."模板匹配参数 " ("Main")) -> ()  [unwired: 2 in, 2 out]
      }
    }
    n148 = call "GetSystemTime.vi"() -> ("date/time string"=→"system time":string)  [unwired: 7 in]
  }
  n149 = call "Release Queue Array.vi"("error in"=w3, "queue in"=w1) -> ("error out"=w2:errorcluster)  [unwired: 2 in, 3 out]
  n150 = call "Release Queue Array.vi"("error in"=w6, "queue in"=w1) -> ("error out"=w9:errorcluster)  [unwired: 2 in, 3 out]
  n151 = call "MergeErrors.vi"("error in 3 (no error)"=w2, "error in 4 (no error)"=w9) -> ("error out"=w8:errorcluster)  [unwired: 6 in]
  n152 = call "ExitAppMode.vi"("error in (no error)"=w8) -> ("error out"=w7:errorcluster)  [unwired: 10 in]
  n153 = call <vilib>:"Clear Errors.vi"("error in (no error)"=w7) -> ()  [unwired: 5 in, 2 out]
